vi "Make SEQ.vi"(0 "Base File Name":string, 4 "Header file data":T1 {"Pixel depth" items=["8 bits", "16 bits", "Float", "Complex", "RGB", "HSL"]; "time of 1st frame, \nsec since 1/1/04" format="%.2f"}, 5 "Acqisition files refnums":refnum<file>[](array[refnum]), 6 "Number of images":u32, 7 "AOI List":u16[][](array[numeric]), 8 "Description":string, 9 "User Info":string="Unknown User", 10 "First image number (start 0)":u32) -> ()   [LabVIEW 2011]
doc: "Saves video data in the \".seq\" format read by PROTO*. Only the temporal and spatial protions of the video specified in the first image number, number of images, and aoi list parameters are saved."
uses:
  Header file data.ctl
  Seq file v 1/Offset table.ctl
  Seq file v 1/Offset.ctl
  Seq file v 1/file number.ctl
panel:
  out "Time table file name":string
  out "SEQ file name":string
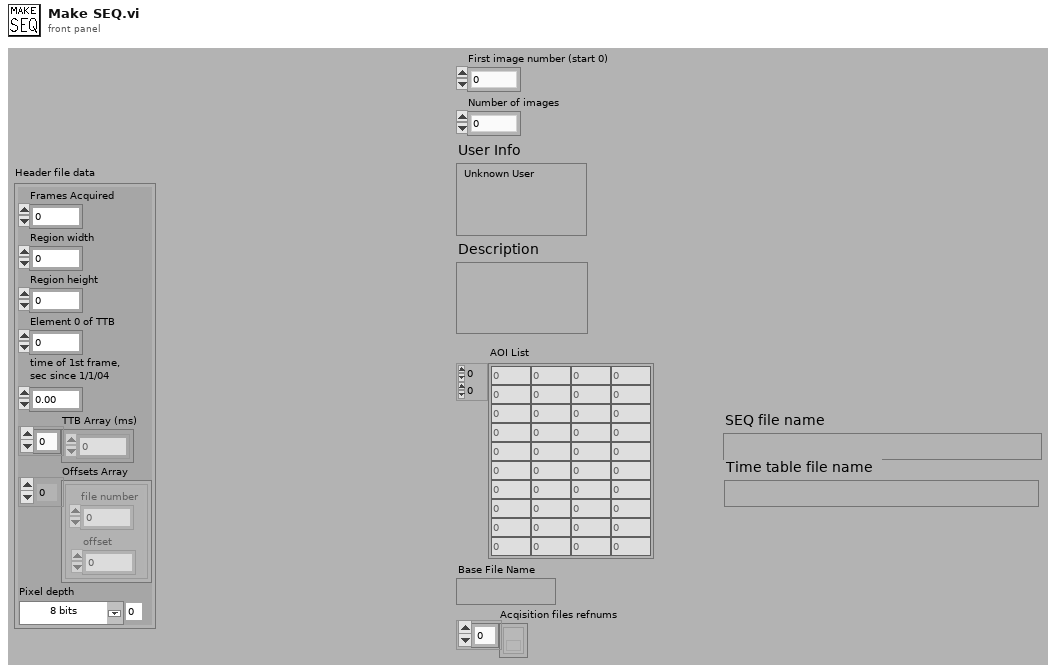
[diagram p1: front panel]
types:
  T1 = typedef "Header file data.ctl" = cluster{"Frames Acquired":u32, "Region width":i32, "Region height":i32, "Element 0 of TTB":u32, "time of 1st frame, \nsec since 1/1/04":dbl, "TTB Array (ms)":u32[], "Offsets Array":T2, "Pixel depth":u32}
  T2 = typedef "Offset table.ctl" = cluster{"offset":T3, "file number":T4}[]
  T3 = typedef "Offset.ctl" = i32
  T4 = typedef "file number.ctl" = u8
  T5 = enum16{"open", "open or create", "create or replace", "create"}
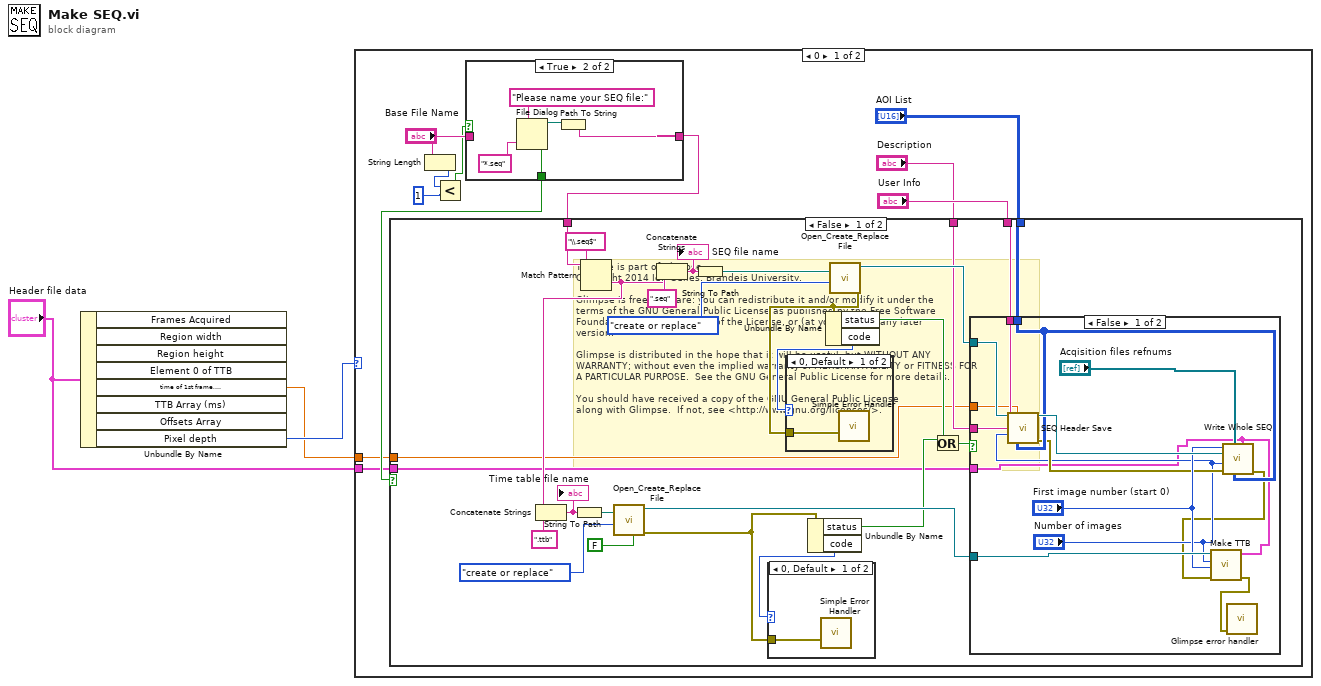
[diagram p0: block diagram]
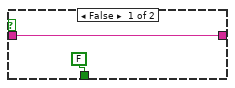
[diagram p6: hidden frame]
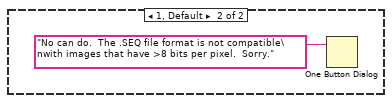
[diagram p7: hidden frame]
diagram:
  # "This file is part of Glimpse. \nCopyright 2014 Jeff Gelles, Brandeis University.    \n\nGlimpse is free software: you can redistribute it and/or modify it under the \nterms of the GNU General Public License as published by the Free Software \nFoundation, either version 3 of the License, or (at your option) any later \nversion.\n\nGlimpse is distributed in the hope that it will be useful, but WITHOUT ANY \nWARRANTY; without even the implied warranty of MERCHANTABILITY or FITNESS FOR \nA PARTICULAR PURPOSE.  See the GNU General Public License for more details.\n\nYou should have received a copy of the GNU General Public License\nalong with Glimpse.  If not, see <http://www.gnu.org/licenses/>."
  n1 = Unbundle By Name("Header file data") -> ("time of 1st frame, \nsec since 1/1/04"=w2:dbl, "Pixel depth"=w3:u32)  [unwired: 6 out]
  n2 = case shown="0" w3 {
    tunnel: w2 -> [w5 _]
    tunnel: "Header file data" -> [w4 _]
    frame 0 {
      n3 = String Length(string="Base File Name") -> (length=w7:i32)
      n4 = Less?(x=w7, y=1) -> (x < y?=w10:bool)
      n5 = case shown="True" w10 {
        tunnel: [w58 w61] -> w14
        tunnel: "Base File Name" -> [w58 _]
        tunnel: [FALSE ("cancelled") w59] -> w8
        frame False {
        }
        frame True {
          n6 = File Dialog(6:"*.seq" ("pattern"), 7:"Please name your SEQ file:" ("prompt")) -> (1:w59:bool, 3:w62:path)  [unwired: 1 in, 6 out]
          n7 = Path To String(path=w62) -> (string=w61:string)
        }
      }
      n8 = case shown="False" w8 {
        tunnel: w14 -> [w38 _]
        tunnel: "User Info" -> [w34 _]
        tunnel: "Description" -> [w33 _]
        tunnel: "AOI List" -> [w28 _]
        tunnel: w5 -> [w16 _]
        tunnel: w4 -> [w15 _]
        frame False {
          n9 = Match Pattern(string=w38, regular expression="\\.seq$") -> (before substring=w29:string)  [unwired: 4 out]
          n10 = Concatenate Strings(w29, ".ttb") -> (w31:string)
          "Time table file name" <- w31
          n11 = String To Path(string=w31) -> (path=w30:path)
          n12 = call <vilib>:"Open_Create_Replace File.vi"("advisory dialog? (display:T)"=FALSE, "function (open:0)"=T5."create or replace", "file path"=w30) -> ("error out"=w19:errorcluster, "refnum"=w23:refnum<file>)  [unwired: 4 in, 3 out]
          n13 = Concatenate Strings(w29, ".seq") -> (w37:string)
          "SEQ file name" <- w37
          n14 = String To Path(string=w37) -> (path=w36:path)
          n15 = Unbundle By Name(w19) -> ("status"=w20:bool, "code"=w22:i32)
          n16 = case shown="0, Default" w22 {
            tunnel: w19 -> [w41 _]
            frame 0, Default {
              n17 = call <vilib>:"Simple Error Handler.vi"("error in (no error)"=w41) -> ()  [unwired: 1 in, 8 out]
            }
            frame 43 {
            }
          }
          n18 = call <vilib>:"Open_Create_Replace File.vi"("function (open:0)"=T5."create or replace", "file path"=w36) -> ("error out"=w24:errorcluster, "refnum"=w35:refnum<file>)  [unwired: 4 in, 4 out]
          n19 = Unbundle By Name(w24) -> ("status"=w26:bool, "code"=w25:i32)
          n20 = case shown="0, Default" w25 {
            tunnel: w24 -> [w42 _]
            frame 0, Default {
              n21 = call <vilib>:"Simple Error Handler.vi"("error in (no error)"=w42) -> ()  [unwired: 1 in, 8 out]
            }
            frame 43 {
            }
          }
          n22 = Or(x=w20, y=w26) -> (x .or. y?=w21:bool)
          n23 = case shown="False" w21 {
            tunnel: w35 -> [w55 _]
            tunnel: w34 -> [w54 _]
            tunnel: w33 -> [w53 _]
            tunnel: w28 -> [w52 _]
            tunnel: w23 -> [w51 _]
            tunnel: w16 -> [w44 _]
            tunnel: w15 -> [w43 _]
            frame False {
              n24 = call "SEQ Header Save.vi"("refnum"=w55, "time of 1st frame, \nsec since 1/1/04"=w44, "User Info"=w54, "Description"=w53, "# of Frames"="Number of images", "AOI List"=w52) -> ("dup refnum"=w56:refnum<file>, "error out"=w48:errorcluster)  [unwired: 1 in, 7 out]
              n25 = call "Write Whole SEQ.vi"("Header file data"=w43, "AOI List"=w52, "Acqisition files refnums"="Acqisition files refnums", "error in"=w48, "Number of images"="Number of images", "SEQ file refnum"=w56, "First image number"="First image number (start 0)") -> ("error out"=w46:errorcluster)  [unwired: 3 out]
              n26 = call "Make TTB.vi"("Header file data"=w43, "error in (no error)"=w46, "first frame number"="First image number (start 0)", "# of frames"="Number of images", "refnum"=w51) -> ("error out"=w45:errorcluster)  [unwired: 2 out]
              n27 = call "Glimpse error handler.vi"("error in"=w45) -> ()  [unwired: 1 in, 6 out]
            }
            frame True {
            }
          }
        }
        frame True {
        }
      }
    }
    frame 1, Default {
      n28 = One Button Dialog(message="No can do.  The .SEQ file format is not compatible\nwith images that have >8 bits per pixel.  Sorry.") -> ()  [unwired: 2 out]
    }
  }
